vi "Test - Run MQTT.vi"() -> ()   [LabVIEW 2020]
uses:
  <vilib>/LabVIEW Open Source Project/MQTT Client/Client class/Client.lvclass/Client.ctl
  <vilib>/LabVIEW Open Source Project/MQTT Connection/MQTT_Base/Base Class/MQTT_Base.lvclass/MQTT_Base.ctl
  92fb48f5-4a4c-4318-8b79-0b24c31d4907.vi
  <vilib>/LabVIEW Open Source Project/MQTT TCP Connection/MQTT_TCP/Connection/TCPConnection.lvclass
  C:/Program Files (x86)/National Instruments/LabVIEW 2020/vi.lib/LabVIEW Open Source Project/MQTT Connection/MQTT_Connection/Connection/Connection.lvclass
  <vilib>/LabVIEW Open Source Project/MQTT Client/Client class/Client.lvclass
  C:/Program Files (x86)/National Instruments/LabVIEW 2020/vi.lib/LabVIEW Open Source Project/MQTT Connection/MQTT_Base/Base Class/MQTT_Base.lvclass
  <vilib>/LabVIEW Open Source Project/MQTT Control Packets/Control Packets/PUBLISH/PUBLISH.lvclass
  <vilib>/LabVIEW Open Source Project/MQTT Connection/MQTT_Base/Base Class/MQTT_Base.lvclass
panel:
  in  "Boolean":bool
  in  "Connection":bool
  in  "Stop Client":bool
  out "Published":bool
  out "Waveform Chart":dbl(graph)
  out "last error":errorcluster
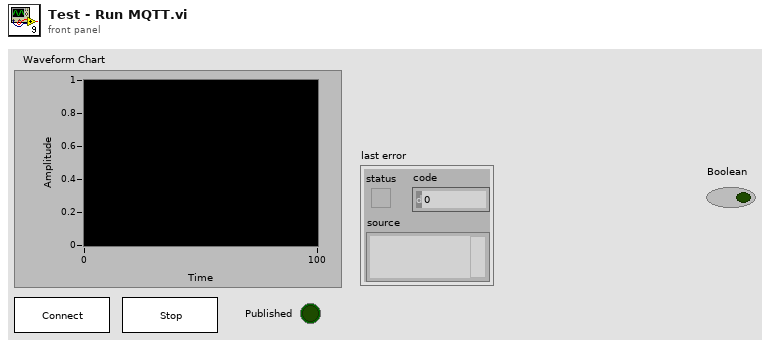
[diagram p1: front panel]
types:
  T1 = typedef "MQTT Client.lvlib/Client.lvclass/Public Events -- cluster.ctl" = cluster{"Connection Status":refnum<user-event>, "Connected":refnum<user-event>, "Application Message":refnum<user-event>}
  T2 = typedef "MQTT Base.lvlib/MQTT_Base.lvclass/Public Events -- cluster.ctl" = cluster{"Stop Event":refnum<user-event>, "Error Event":refnum<user-event>, "Inbound Message":refnum<user-event>}
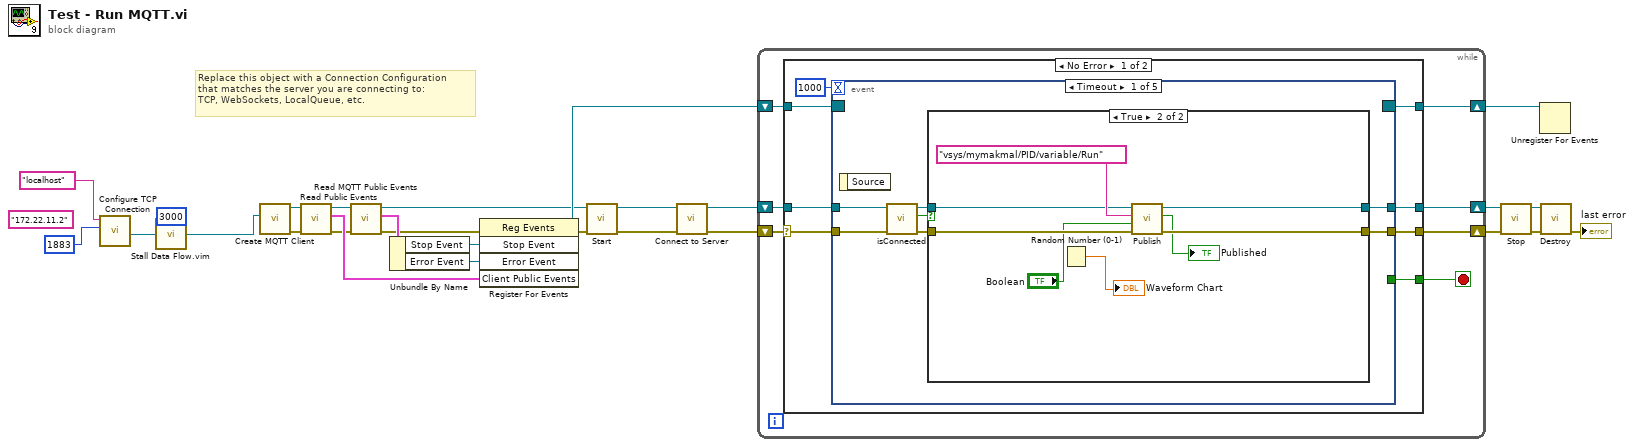
[diagram p0: block diagram]
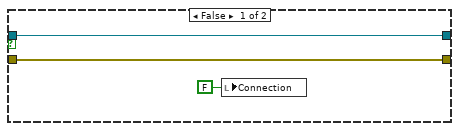
[diagram p2: hidden frame]
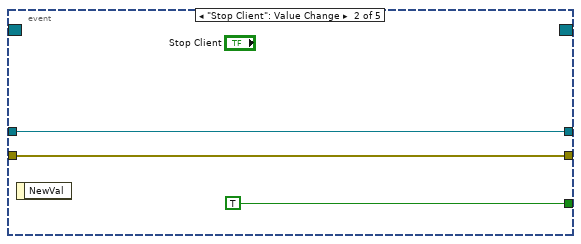
[diagram p3: hidden frame]
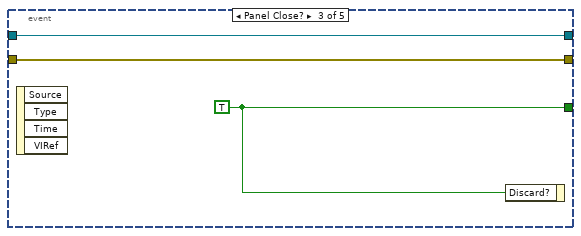
[diagram p4: hidden frame]
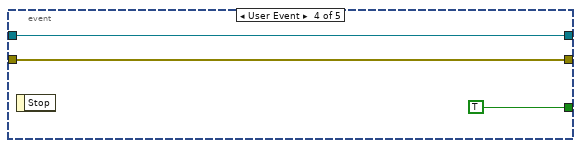
[diagram p5: hidden frame]
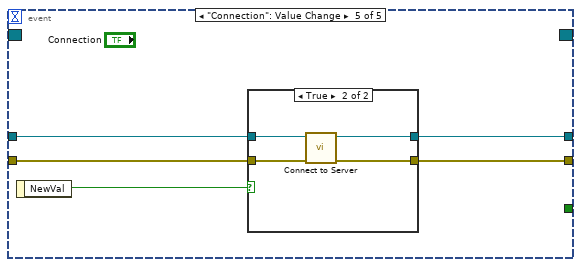
[diagram p6: hidden frame]
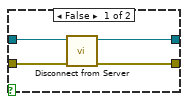
[diagram p7: hidden frame]
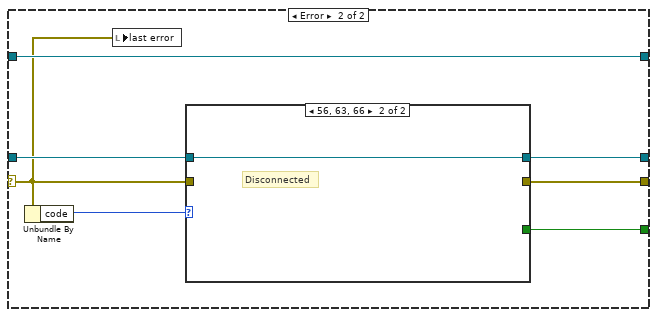
[diagram p8: hidden frame]
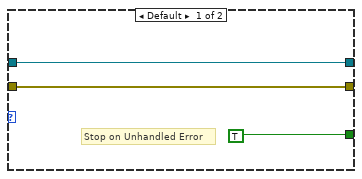
[diagram p9: hidden frame]
diagram:
  (unwired) "172.22.11.2" ("address (localhost)")
  # "Replace this object with a Connection Configuration\nthat matches the server you are connecting to:\nTCP, WebSockets, LocalQueue, etc."
  n1 = call <vilib>:"Configure TCP Connection.vi"("remote port (80)"=u16 1883, "address (localhost)"="localhost") -> ("TCPConnection"=w7:refnum<class "TCPConnection.lvclass">)  [unwired: 8 in, 1 out]
  n2 = call "Stall Data Flow.vim"("value in"=w7, "milliseconds to wait"=u32 3000) -> ("value out"=w6:refnum<class "TCPConnection.lvclass">)  [unwired: 1 out]
  n3 = call <vilib>:"Create MQTT Client.vi"("Connection Configuration"=w6) -> ("error out"=w12:errorcluster, "Client out"=w10:refnum<class "Client.lvclass">)  [unwired: 9 in]
  n4 = call <vilib>:"Read Public Events.vi"("error in (no error)"=w12, "Client in"=w10) -> ("error out"=w13:errorcluster, "Client Public Events"=w15:T1, "Client out"=w11:refnum<class "Client.lvclass">)  [unwired: 7 in]
  n5 = call <vilib>:"Read MQTT Public Events.vi"("error in (no error)"=w13, "MQTT_Base in"=w11) -> ("error out"=w14:errorcluster, "MQTT Public Events"=w22:T2, "MQTT_Base out"=w17:refnum<class "Client.lvclass">)  [unwired: 7 in]
  n6 = Unbundle By Name(w22) -> ("Stop Event"=w20:refnum<user-event>, "Error Event"=w21:refnum<user-event>)
  n7 = register-events(error in=w14, w20, w21, w15) -> (reference out=w18:refnum<event-registration>, error out=w16:errorcluster)  [unwired: 1 in]
  n8 = call <vilib>:"Start.vi"("error in (no error)"=w16, "MQTT_Base in"=w17) -> ("error out"=w2:errorcluster, "MQTT_Base out"=w4:refnum<class "Client.lvclass">)  [unwired: 7 in, 1 out]
  n9 = call <vilib>:"Connect to Server.vi"("error in (no error)"=w2, "Client in"=w4) -> ("error out"=w1:errorcluster, "Client out"=w3:refnum<class "Client.lvclass">)  [unwired: 6 in, 2 out]
  n10 = while {
    shift-right: [w33] -> w19
    shift-left: w18 -> [w34]
    shift-right: [w30] -> w24
    shift-left: w3 -> [w31]
    shift-right: [w32] -> w26
    shift-left: w1 -> [w28]
    stop <- w29 stop-if-true
    n11 = case shown="No Error" w28 {
      selector: w28 -> [w35 w83]
      tunnel: w34 -> [w42 w89]
      tunnel: [w41 w89] -> w33
      tunnel: [w40 w85] -> w32
      tunnel: w31 -> [w38 w87]
      tunnel: [w37 w86] -> w30
      tunnel: [w36 w84] -> w29
      frame No Error {
        n12 = event shown="[0] Timeout" {
          selector: w42 -> [_ _ _ _ _]
          dyn-events: [_ _ _ _ _] -> w41
          timeout: 1000 -> [_ _ _ _ _]
          tunnel: w35 -> [w45 w62 w64 w69 w70]
          tunnel: [w48 w62 w64 w69 w71] -> w40
          tunnel: [_ TRUE w66 TRUE _] -> w36
          tunnel: w38 -> [w47 w63 w65 w67 w74]
          tunnel: [w49 w63 w65 w67 w72] -> w37
          event Timeout {
            n13 = event-data() -> ()  [unwired: 1 in, 1 out]
            n14 = call <vilib>:"isConnected.vi"("error in (no error)"=w45, "Client in"=w47) -> ("error out"=w44:errorcluster, "connected"=w43:bool, "Client out"=w46:refnum<class "Client.lvclass">)  [unwired: 7 in]
            n15 = case shown="True" w43 {
              tunnel: [w52 w59] -> w49
              tunnel: [w51 w58] -> w48
              tunnel: w46 -> [w52 w55]
              tunnel: w44 -> [w51 w54]
              frame False {
                n16 = local write "Connection"(FALSE ("Connection")) -> ()
              }
              frame True {
                n17 = Random Number (0-1)() -> (number: 0 to 1=→"Waveform Chart":dbl)
                n18 = call <vilib>:"Publish.vi"("error in (no error)"=w54, "Payload"="Boolean", "Topic Name (empty: Payload name)"="vsys/mymakmal/PID/variable/Run", "Client in"=w55) -> ("error out"=w58:errorcluster, "Published"=→"Published":bool, "Client out"=w59:refnum<class "Client.lvclass">)  [unwired: 5 in]
              }
            }
          }
          event "Stop Client": Value Change {
            n19 = event-data() -> ()  [unwired: 1 in, 1 out]
          }
          event Panel Close? {
            w66 = TRUE
            n20 = event-data() -> ()  [unwired: 1 in, 4 out]
            n21 = event-data("Discard?"=w66) -> ()  [unwired: 1 in, 1 out]
          }
          event User Event {
            n22 = event-data() -> ()  [unwired: 1 in, 1 out]
          }
          event "Connection": Value Change {
            n23 = event-data() -> ("NewVal"=w73:bool)  [unwired: 1 in]
            n24 = case shown="True" w73 {
              tunnel: w74 -> [w78 w82]
              tunnel: [w77 w79] -> w72
              tunnel: [w76 w80] -> w71
              tunnel: w70 -> [w75 w81]
              frame False {
                n25 = call <vilib>:"Disconnect from Server.vi"("error in (no error)"=w75, "Client in"=w78) -> ("error out"=w76:errorcluster, "Client out"=w77:refnum<class "Client.lvclass">)  [unwired: 7 in, 1 out]
              }
              frame True {
                n26 = call <vilib>:"Connect to Server.vi"("error in (no error)"=w81, "Client in"=w82) -> ("error out"=w80:errorcluster, "Client out"=w79:refnum<class "Client.lvclass">)  [unwired: 6 in, 2 out]
              }
            }
          }
        }
      }
      frame Error {
        n27 = Unbundle By Name(w83) -> ("code"=w88:i32)
        n28 = local write "last error"(w83) -> ()
        n29 = case shown="56, 63, 66" w88 {
          tunnel: w87 -> [w92 w93]
          tunnel: [w92 w93] -> w86
          tunnel: w83 -> [w91 _]
          tunnel: [w91 _] -> w85
          tunnel: [TRUE _] -> w84
          frame Default {
            # "Stop on Unhandled Error"
          }
          frame 56, 63, 66 {
            # "Disconnected"
          }
        }
      }
    }
  }
  n30 = call <vilib>:"Stop.vi"("error in (no error)"=w26, "MQTT_Base in"=w24) -> ("error out"=w25:errorcluster, "MQTT_Base out"=w23:refnum<class "Client.lvclass">)  [unwired: 7 in, 1 out]
  n31 = Unregister For Events(event registration refnum=w19) -> ()  [unwired: 1 in, 1 out]
  n32 = call <vilib>:"Destroy.vi"("error in (no error)"=w25, "MQTT_Base in"=w23) -> ("error out"=→"last error":errorcluster)  [unwired: 8 in, 1 out]
